vi "File_Module.vi"(7 "Command":T4, 8 "error in (no error)":errorcluster, 9 "Datos.Ensayo":T3={"Tiempo (min)"=1.0, "Temperatura.ext, C"=0.0, "Humedad.Rel.ext, f1"=0.0, "Temp.pt100.1, C"=1.0, "Temp.pt100.2, C"=1.0, "Temp.pt100.3, C"=0.0, "Temp.pt100.4, C"=0.0, "Temp.termopar.5, C"=0.0, "Temp.termopar.6, C"=0.0, "Humedad.rel.3, f1"=0.0, "Humedad.rel.4, f1"=0.0, "Presion.dif, Pa"=0.0, "P116.set.temp, C"=0.0, "P116.temperatura, C"=0.0, "P116.output, %"=0.0, "P116.output, W"=0.0, "Q.set.caudal, g/s"=0.0, "Q.caudal, g/s"=0.0, "Agua.evapor, g/s"=0.0, "Humedad.lecho, f1"=0.0, "Q.aire.seco, W"=0.0, "Q.evaporacion, W"=0.0, "Porosidad, "=0.0, "Vel.a.lecho, m/s"=0.0, "Vel.min.fluido, m/s"=0.0, "Vel.arrastre, m/s"=0.0} {"Porosidad," format="%.2f"; "Vel.arrastre, m/s" format="%.2f"; "Vel.min.fluido, m/s" format="%.2f"; "Vel.a.lecho, m/s" format="%.2f"; "Q.evaporacion, W" format="%.2f"; "Q.aire.seco, W" format="%.2f"; "Humedad.lecho, f1" format="%.2f"; "Temperatura.ext, C" format="%.2f"; "Humedad.Rel.ext, f1" format="%.2f"; "Q.set.caudal, g/s" format="%.2f"; "Temp.termopar.6, C" format="%.2f"; "Temp.termopar.5, C" format="%.2f"; "P116.output, W" format="%.2f"; "Agua.evapor, g/s" format="%.2f"; "Humedad.rel.3, f1" format="%.2f"; "Temp.pt100.4, C" format="%.2f"; "Temp.pt100.3, C" format="%.2f"; "Q.caudal, g/s" format="%.2f"; "Humedad.rel.4, f1" format="%.2f"; "P116.temperatura, C" format="%.2f"; "P116.set.temp, C" format="%.2f"; "P116.output, %" format="%.2f"; "Temp.pt100.2, C" format="%.2f"; "Presion.dif, Pa" format="%.2f"; "Temp.pt100.1, C" format="%.2f"; "Tiempo (min)" format="%.2f"}, 10 "Datos.Lecho":T1={"Clasificacion"="Grueso (2,5<Dp<4", "Masa, g"=500.0, "Altura, cm"=45.0, "Diam_part, mm"=5.0, "Dens_part, g/cm3"=1.0, "Hum_ini, %"=60.0, "Temp_ini, C"=25.0} {"Hum_ini, %" format="%.2f"; "Temp_ini, C" format="%.2f"; "Masa, g" format="%.2f"; "Altura, cm" format="%.2f"; "Diam_part, mm" format="%.2f"; "Dens_part, g/cm3" format="%.2f"}, 11 "Constantes.Ensayo":T2={"Num.Ensayo"=0, "Diam_reactor, cm"=1.0, "Resistencia, ohm"=50.0, "Voltaje_resist, vac"=230.0, "Hum_ext, %"=0.0, "Vel.min_fluido, m/s"=0.0, "Vel_arrastre, m/s"=0.0, "SET Caudal_vent, g/s"=5.0} {"Vel_arrastre, m/s" format="%.2f"; "SET Caudal_vent, g/s" format="%.2f"; "Diam_reactor, cm" format="%.2f"; "Resistencia, ohm" format="%.2f"; "Voltaje_resist, vac" format="%.2f"; "Hum_ext, %" format="%.2f"; "Vel.min_fluido, m/s" format="%.2f"}) -> (0 "error out":errorcluster, 2 "selected path":path)   [LabVIEW 2017]
uses:
  File_Module Control.ctl
  Typedefs/SECADO_datos.Ensayo--Cluster.ctl
  Typedefs/SECADO_constantes.Ensayo--Cluster.ctl
  Typedefs/SECADO_datos.Lecho--Cluster.ctl
panel:
  out "Cabeceras":string[](array[string])
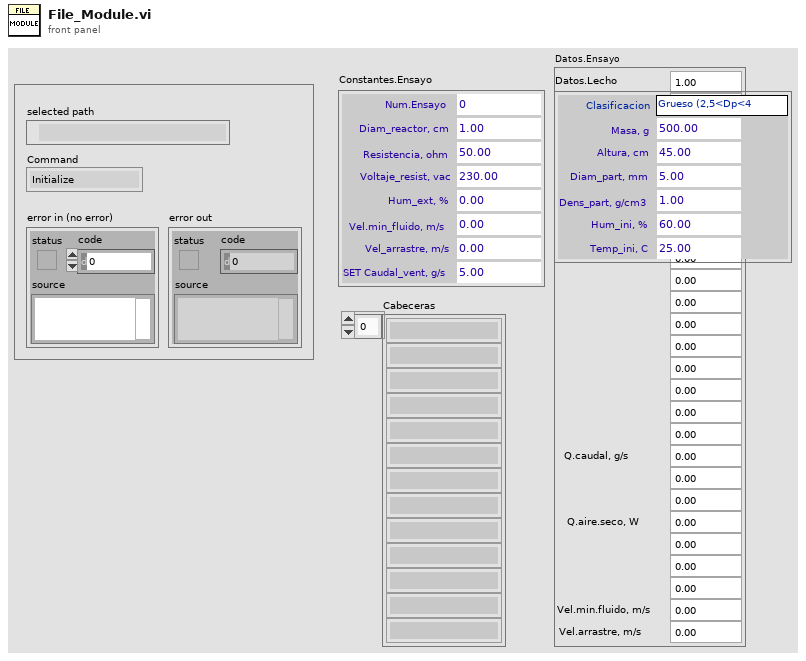
[diagram p1: front panel]
types:
  T1 = typedef "SECADO_datos.Lecho--Cluster.ctl" = cluster{"Clasificacion":string, "Masa, g":dbl, "Altura, cm":dbl, "Diam_part, mm":dbl, "Dens_part, g/cm3":dbl, "Hum_ini, %":dbl, "Temp_ini, C":dbl}
  T2 = typedef "SECADO_constantes.Ensayo--Cluster.ctl" = cluster{"Num.Ensayo":i32, "Diam_reactor, cm":dbl, "Resistencia, ohm":dbl, "Voltaje_resist, vac":dbl, "Hum_ext, %":dbl, "Vel.min_fluido, m/s":dbl, "Vel_arrastre, m/s":dbl, "SET Caudal_vent, g/s":dbl}
  T3 = typedef "SECADO_datos.Ensayo--Cluster.ctl" = cluster{"Tiempo (min)":dbl, "Temperatura.ext, C":dbl, "Humedad.Rel.ext, f1":dbl, "Temp.pt100.1, C":dbl, "Temp.pt100.2, C":dbl, "Temp.pt100.3, C":dbl, "Temp.pt100.4, C":dbl, "Temp.termopar.5, C":dbl, "Temp.termopar.6, C":dbl, "Humedad.rel.3, f1":dbl, "Humedad.rel.4, f1":dbl, "Presion.dif, Pa":dbl, "P116.set.temp, C":dbl, "P116.temperatura, C":dbl, "P116.output, %":dbl, "P116.output, W":dbl, "Q.set.caudal, g/s":dbl, "Q.caudal, g/s":dbl, "Agua.evapor, g/s":dbl, "Humedad.lecho, f1":dbl, "Q.aire.seco, W":dbl, "Q.evaporacion, W":dbl, "Porosidad, ":dbl, "Vel.a.lecho, m/s":dbl, "Vel.min.fluido, m/s":dbl, "Vel.arrastre, m/s":dbl}
  T4 = typedef "File_Module Control.ctl" = enum16{"Initialize", "Save Head", "Save Data", "Shutdown"}
  T5 = enum16{"open", "replace", "create", "open or create", "replace or create", "replace or create with confirmation"}
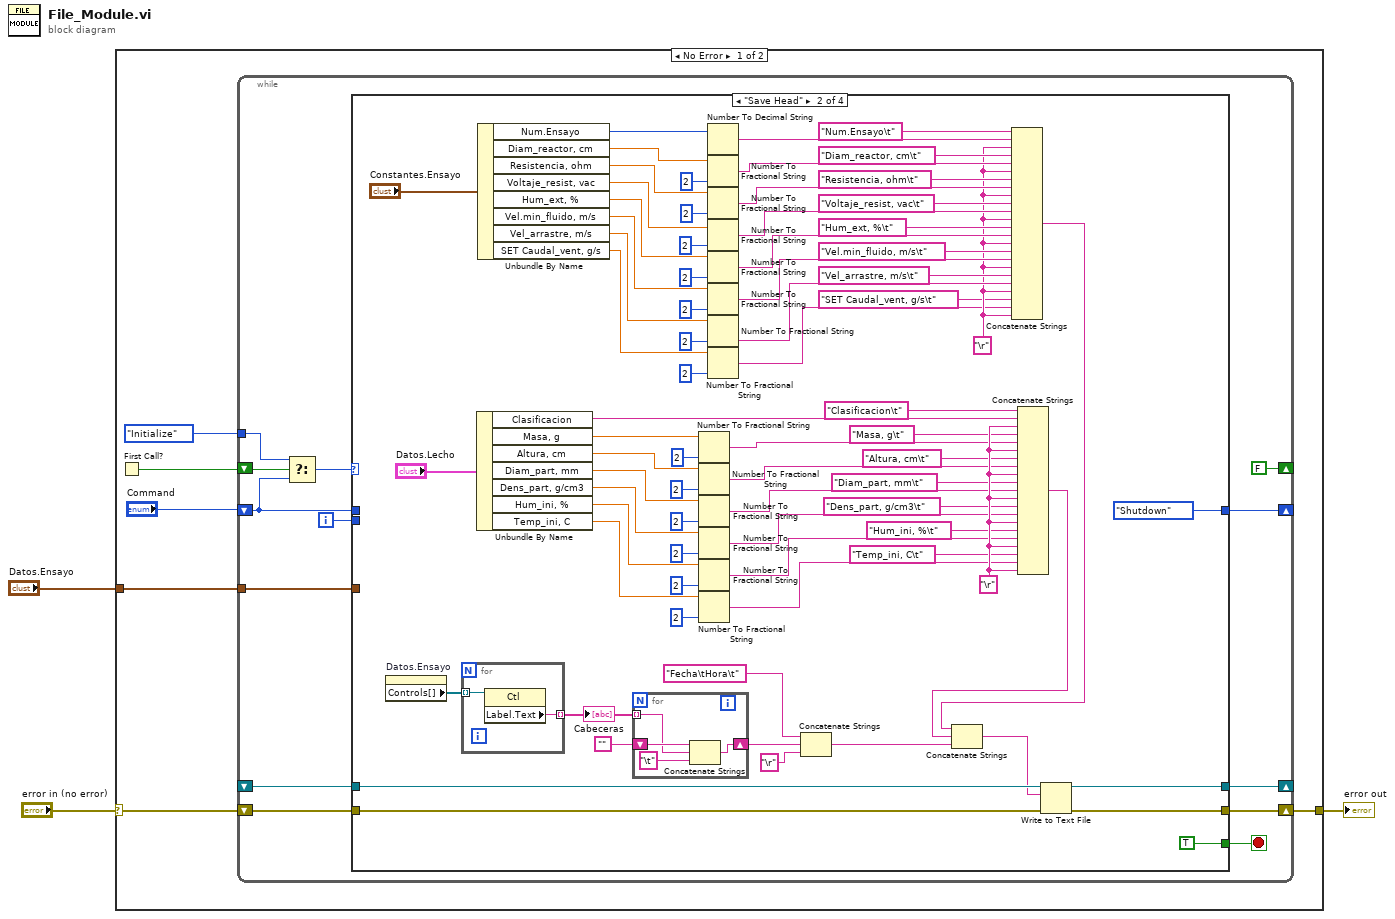
[diagram p0: block diagram]
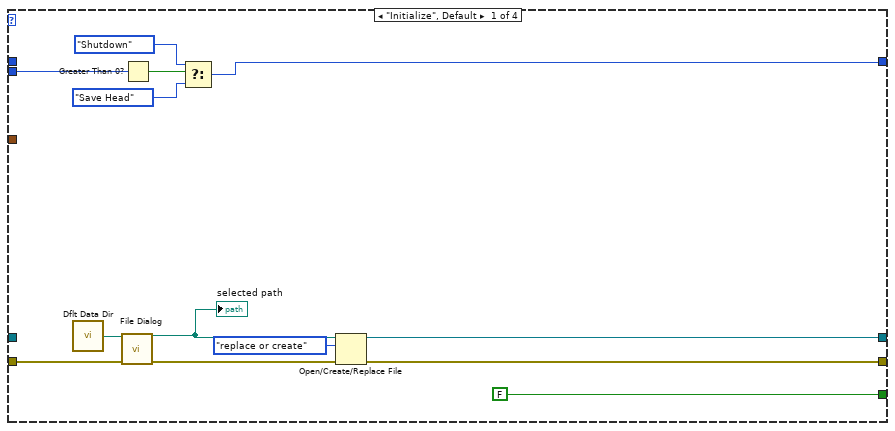
[diagram p2: hidden frame]
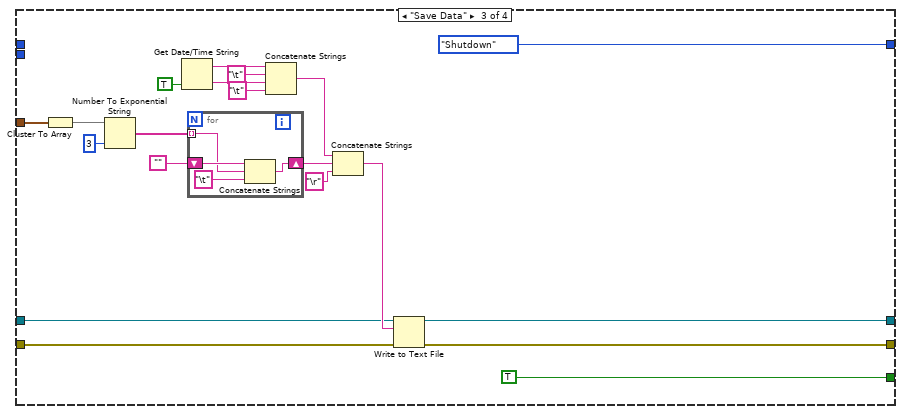
[diagram p3: hidden frame]
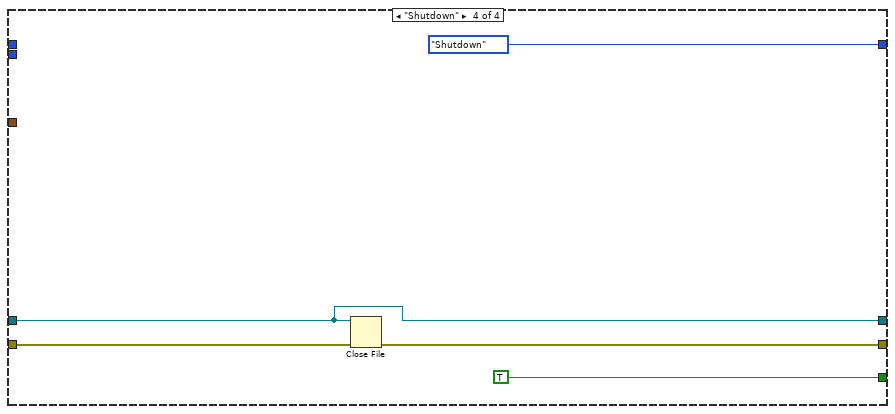
[diagram p4: hidden frame]
diagram:
  n1 = case shown="No Error" "error in (no error)" {
    selector: "error in (no error)" -> [w7 w148]
    tunnel: [w6 w148] -> w2
    tunnel: "Datos.Ensayo" -> [w4 _]
    frame No Error {
      n2 = First Call?() -> (First Call?: T/F=w9:bool)
      n3 = while {
        shift-right: [w14] -> _
        shift-left: "Command" -> [w15]
        shift-right: [w17] -> w6
        shift-left: w7 -> [w18]
        shift-right: [FALSE ("First Call?: T/F")] -> _
        shift-left: w9 -> [w22]
        tunnel: File_Module_Control."Initialize" ("t") -> [w21]
        shift-right: [w11] -> _
        shift-left: _ -> [w12]
        tunnel: w4 -> [w10]
        i -> [w13]
        stop <- w19 stop-if-true
        n4 = Select(t=w21, s=w22, f=w15) -> (s? t:f=w20:T4)
        n5 = case shown="\"Save Head\"" w20 {
          tunnel: [FALSE TRUE TRUE TRUE] -> w19
          tunnel: w18 -> [w28 w108 w129 w145]
          tunnel: [w24 w107 w128 w144] -> w17
          tunnel: w15 -> [_ _ _ _]
          tunnel: [w34 File_Module_Control."Shutdown" ("t") File_Module_Control."Shutdown" File_Module_Control."Shutdown"] -> w14
          tunnel: w13 -> [w32 _ _ _]
          tunnel: w12 -> [_ w110 w125 w143]
          tunnel: [w23 w109 w127 w143] -> w11
          tunnel: w10 -> [_ _ w131 _]
          frame "Initialize", Default {
            n6 = call <vilib>:"Dflt Data Dir.vi"() -> ("App:Default Data Directory"=w29:path)
            n7 = call "File Dialog"("start path"=w29, "error in"=w28) -> ("selected path"=w26:path, "error out"=w25:errorcluster)  [unwired: 10 in, 2 out]
            "selected path" <- w26
            n8 = Greater Than 0?(x=w32) -> (x > 0?=w31:bool)
            n9 = Select(t=File_Module_Control."Shutdown", s=w31, f=File_Module_Control."Save Head" ("t")) -> (s? t:f=w34:T4)
            n10 = Open/Create/Replace File(file path (use dialog)=w26, error in=w25, operation (0:open)=T5."replace or create") -> (refnum out=w23:refnum<file>, error out=w24:errorcluster)  [unwired: 3 in, 1 out]
          }
          frame "Save Head" {
            w64 = "\r" ("string")
            w67 = "\r" ("string")
            n11 = property on="Datos.Ensayo" class="Clust (strict)"() -> ("Controls[]"=w106:refnum<vi>[])  [unwired: 2 in, 2 out]
            n12 = for {
              tunnel: w106 -> [w118] mode=indexing
              tunnel: [w117] -> w101 mode=indexing
              n13 = property class="Ctl"(reference=w118) -> ("Label.Text"=w117:string)  [unwired: 1 in, 2 out]
            }
            "Cabeceras" <- w101
            n14 = Unbundle By Name("Datos.Lecho") -> ("Clasificacion"=w56:string, "Masa, g"=w50:dbl, "Altura, cm"=w49:dbl, "Diam_part, mm"=w47:dbl, "Dens_part, g/cm3"=w46:dbl, "Hum_ini, %"=w45:dbl, "Temp_ini, C"=w44:dbl)
            n15 = Unbundle By Name("Constantes.Ensayo") -> ("Num.Ensayo"=w89:i32, "Diam_reactor, cm"=w80:dbl, "Resistencia, ohm"=w79:dbl, "Voltaje_resist, vac"=w78:dbl, "Hum_ext, %"=w77:dbl, "Vel.min_fluido, m/s"=w76:dbl, "Vel_arrastre, m/s"=w75:dbl, "SET Caudal_vent, g/s"=w74:dbl)
            n16 = for {
              tunnel: w101 -> [w115] mode=indexing
              shift-right: [w114] -> w105
              shift-left: "" -> [w116]
              n17 = Concatenate Strings(w116, w115, "\t" ("string")) -> (w114:string)
            }
            n18 = Number To Fractional String(number=w50, precision (6)=i16 2) -> (F-format string=w43:string)  [unwired: 2 in]
            n19 = Number To Fractional String(number=w49, precision (6)=i16 2) -> (F-format string=w42:string)  [unwired: 2 in]
            n20 = Number To Fractional String(number=w47, precision (6)=i16 2) -> (F-format string=w41:string)  [unwired: 2 in]
            n21 = Number To Fractional String(number=w46, precision (6)=i16 2) -> (F-format string=w40:string)  [unwired: 2 in]
            n22 = Number To Fractional String(number=w45, precision (6)=i16 2) -> (F-format string=w39:string)  [unwired: 2 in]
            n23 = Number To Fractional String(number=w44, precision (6)=i16 2) -> (F-format string=w38:string)  [unwired: 2 in]
            n24 = Number To Decimal String(number=w89) -> (decimal integer string=w88:string)  [unwired: 1 in]
            n25 = Number To Fractional String(number=w80, precision (6)=i16 2) -> (F-format string=w73:string)  [unwired: 2 in]
            n26 = Number To Fractional String(number=w79, precision (6)=i16 2) -> (F-format string=w72:string)  [unwired: 2 in]
            n27 = Number To Fractional String(number=w78, precision (6)=i16 2) -> (F-format string=w71:string)  [unwired: 2 in]
            n28 = Number To Fractional String(number=w77, precision (6)=i16 2) -> (F-format string=w70:string)  [unwired: 2 in]
            n29 = Number To Fractional String(number=w76, precision (6)=i16 2) -> (F-format string=w69:string)  [unwired: 2 in]
            n30 = Number To Fractional String(number=w75, precision (6)=i16 2) -> (F-format string=w68:string)  [unwired: 2 in]
            n31 = Number To Fractional String(number=w74, precision (6)=i16 2) -> (F-format string=w65:string)  [unwired: 2 in]
            n32 = Concatenate Strings("Fecha\tHora\t" ("string"), w105, "\r" ("string")) -> (w92:string)
            n33 = Concatenate Strings("Num.Ensayo\t" ("string"), w88, w67, "Diam_reactor, cm\t" ("string"), w73, w67, "Resistencia, ohm\t" ("string"), w72, w67, "Voltaje_resist, vac\t" ("string"), w71, w67, "Hum_ext, %\t" ("string"), w70, w67, "Vel.min_fluido, m/s\t" ("string"), w69, w67, "Vel_arrastre, m/s\t" ("string"), w68, w67, "SET Caudal_vent, g/s\t" ("string"), w65, w67) -> (w37:string)
            n34 = Concatenate Strings("Clasificacion\t" ("string"), w56, w64, "Masa, g\t" ("string"), w43, w64, "Altura, cm\t" ("string"), w42, w64, "Diam_part, mm\t" ("string"), w41, w64, "Dens_part, g/cm3\t" ("string"), w40, w64, "Hum_ini, %\t" ("string"), w39, w64, "Temp_ini, C\t" ("string"), w38, w64) -> (w36:string)
            n35 = Concatenate Strings(w37, w36, w92) -> (w91:string)
            n36 = Write to Text File(file (use dialog)=w110, text=w91, error in=w108) -> (refnum out=w109:refnum<file>, error out=w107:errorcluster)  [unwired: 1 in, 1 out]
          }
          frame "Save Data" {
            n37 = Cluster To Array(cluster=w131) -> (array=w132:dbl[])
            n38 = Number To Exponential String(number=w132, precision (6)=i16 3) -> (E-format string=w130:string[])  [unwired: 2 in]
            n39 = Get Date/Time String(want seconds? (F)=TRUE) -> (date string=w121:string, time string=w120:string)  [unwired: 2 in]
            n40 = for {
              tunnel: w130 -> [w141] mode=indexing
              shift-right: [w140] -> w136
              shift-left: "" -> [w142]
              n41 = Concatenate Strings(w142, w141, "\t" ("string")) -> (w140:string)
            }
            n42 = Concatenate Strings(w121, "\t" ("string"), w120, "\t" ("string")) -> (w124:string)
            n43 = Concatenate Strings(w124, w136, "\r" ("string")) -> (w126:string)
            n44 = Write to Text File(file (use dialog)=w125, text=w126, error in=w129) -> (refnum out=w127:refnum<file>, error out=w128:errorcluster)  [unwired: 1 in, 1 out]
          }
          frame "Shutdown" {
            n45 = Close File(refnum=w143, error in=w145) -> (error out=w144:errorcluster)  [unwired: 1 out]
          }
        }
      }
    }
    frame Error {
    }
  }
  "error out" <- w2
